vi "Read XNET.vi"(8 "error in":errorcluster, 11 "PCAN in":refnum<class "PCAN.lvclass">) -> (0 "error out":errorcluster, 3 "PCAN out":refnum<class "PCAN.lvclass">)   [LabVIEW 2024, in "PCAN.lvclass"]
uses:
  PCAN.lvclass
  D:/git/HAL/HAL/Configurations/CFG Base/CFG Base.lvclass
  Configurations/CFG Base/CFG Base.lvclass/CFG Base.ctl
  PCAN.lvclass/PCAN.ctl
  <vilib>/xnet/xnet.llb/XNET Frame Type CAN.ctl
  <vilib>/xnet/xnet.llb/XNET Convert (Frame CAN to Signal).vi
  Configurations/CFG Base/CFG Base.lvclass
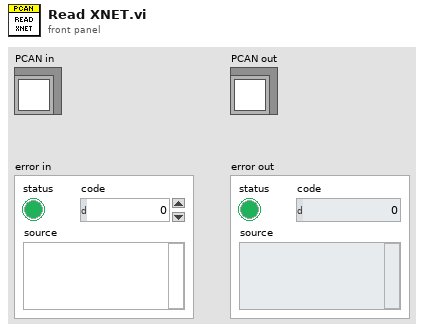
[diagram p1: front panel]
types:
  T1 = typedef "TPCANHandle.ctl" = enum16{"PCAN_NONEBUS  0x000", "PCAN_ISABUS1  0x21", "PCAN_ISABUS2  0x22", "PCAN_ISABUS3  0x23", "PCAN_ISABUS4  0x24", "PCAN_ISABUS5  0x25", "PCAN_ISABUS6  0x26", "PCAN_ISABUS7  0x27", "PCAN_ISABUS8  0x28", "PCAN_DNGBUS1  0x31", "PCAN_PCIBUS1  0x41", "PCAN_PCIBUS1  0x42", "PCAN_PCIBUS1  0x43", "PCAN_PCIBUS1  0x44", "PCAN_PCIBUS1  0x45", "PCAN_PCIBUS1  0x46", "PCAN_PCIBUS1  0x47", "PCAN_PCIBUS1  0x48", "PCAN_PCIBUS1  0x409", "PCAN_PCIBUS1  0x40A", "PCAN_PCIBUS1  0x40B", "PCAN_PCIBUS1  0x40C", "PCAN_PCIBUS1  0x40D", "PCAN_PCIBUS1  0x40E", "PCAN_PCIBUS1  0x40F", "PCAN_PCIBUS1  0x410", "PCAN_USBBUS1  0x51", "PCAN_USBBUS2  0x52", "PCAN_USBBUS3  0x53", "PCAN_USBBUS4  0x54", "PCAN_USBBUS5  0x55", "PCAN_USBBUS6  0x56", "PCAN_USBBUS7  0x57", "PCAN_USBBUS8  0x58", "PCAN_USBBUS9  0x509", "PCAN_USBBUS10  0x50A", "PCAN_USBBUS11  0x50B", "PCAN_USBBUS12  0x50C", "PCAN_USBBUS13  0x50D", "PCAN_USBBUS14  0x50E", "PCAN_USBBUS15  0x50F", "PCAN_USBBUS16  0x510", "PCAN_PCCBUS1  0x61", "PCAN_PCCBUS2  0x62", "PCAN_LANBUS1  0x801", "PCAN_LANBUS2  0x802", "PCAN_LANBUS3  0x803", "PCAN_LANBUS4  0x804", "PCAN_LANBUS5  0x805", "PCAN_LANBUS6  0x806", "PCAN_LANBUS7  0x807", "PCAN_LANBUS8  0x808", "PCAN_LANBUS9  0x809", "PCAN_LANBUS10  0x80A", "PCAN_LANBUS11  0x80B", "PCAN_LANBUS12  0x80C", "PCAN_LANBUS13  0x80D", "PCAN_LANBUS14  0x80E", "PCAN_LANBUS15  0x80F", "PCAN_LANBUS16  0x810"}
  T2 = typedef "TPCANTimestamp.ctl" = cluster{"millis overflow":u16, "millis ":u32, "micros":u16}
  T3 = typedef "CAN MSG Cluster.ctl" = cluster{"ID":u32, "MSG type":u8, "DLC":u8, "DATA":u8[]}
  T4 = typedef "XNET Frame Type CAN.ctl" = u8
  T5 = cluster{"timestamp":timestamp, "payload":u8[], "identifier":u32, "type":T4, "extended?":bool, "echo?":bool}
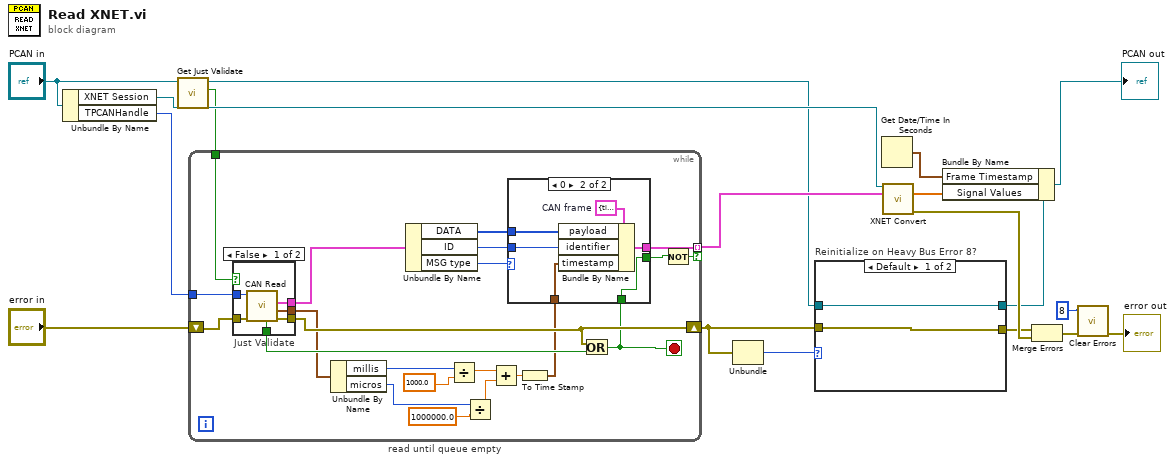
[diagram p0: block diagram]
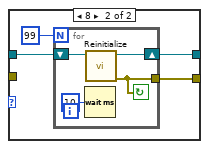
[diagram p2: hidden frame]
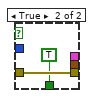
[diagram p3: hidden frame]
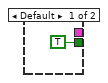
[diagram p4: hidden frame]
diagram:
  n1 = Unbundle By Name("PCAN in") -> ("XNET Session"=w16:refnum<k21>, "TPCANHandle"=w15:T1)
  n2 = call "Get Just Validate.vi"("CFG Base in"="PCAN in") -> ("Just Validate"=w2:bool, "CFG Base out"=w3:refnum<class "PCAN.lvclass">)  [unwired: 9 in]
  n3 = while "read until queue empty" {
    tunnel: w15 -> [w40]
    shift-right: [w37] -> w13
    shift-left: "error in" -> [w39]
    tunnel: [w23] -> w17 mode=indexing if=w36
    tunnel: w2 -> [w19]
    stop <- w20 stop-if-true
    n4 = case "Just Validate" shown="False" w19 {
      tunnel: w40 -> [w46 _]
      tunnel: w39 -> [w45 w48]
      tunnel: [w44 TRUE ("rcv queue empty")] -> w38
      tunnel: [w43 w48] -> w37
      tunnel: [w42 _] -> w35
      tunnel: [w41 _] -> w32
      frame False {
        n5 = call <instrlib>:"CAN Read.vi"("error in (no error)"=w45, "TPCANHandle"=w46) -> ("error out"=w43:errorcluster, "TPCANTimestamp out"=w41:T2, "CAN_Message out"=w42:T3, "rcv queue empty"=w44:bool)  [unwired: 5 in, 1 out]
      }
      frame True {
      }
    }
    n6 = Unbundle By Name(w32) -> ("millis"=w31:u32, "micros"=w29:u16)
    n7 = Unbundle By Name(w35) -> ("DATA"=w34:u8[], "ID"=w33:u32, "MSG type"=w22:u8)
    n8 = Divide(x=w31, y=1000.0) -> (x/y=w25:dbl)
    n9 = Divide(x=w29, y=1000000.0) -> (x/y=w26:dbl)
    n10 = Add(x=w25, y=w26) -> (x+y=w27:dbl)
    n11 = To Time Stamp(1:w27) -> (0:w24:timestamp)
    n12 = Or(x=w37, y=w38) -> (x .or. y?=w20:bool)
    n13 = case shown="0" w22 {
      tunnel: w34 -> [_ w54]
      tunnel: w33 -> [_ w53]
      tunnel: w24 -> [_ w52]
      tunnel: [_ w51] -> w23
      tunnel: [TRUE w50] -> w21
      tunnel: w20 -> [_ w50]
      frame Default {
      }
      frame 0 {
        w55 = T5 {"timestamp"=timestamp(0 s since 1904-01-01), "payload"=[], "identifier"=0, "type"=0, "extended?"=FALSE, "echo?"=FALSE}  # CAN frame
        n14 = Bundle By Name(cluster=w55, "payload"=w54, "identifier"=w53, "timestamp"=w52) -> (w51:T5)
      }
    }
    n15 = Not(x=w21) -> (.not. x?=w36:bool)
  }
  n16 = Unbundle(w13) -> ("code"=w14:i32)  [unwired: 2 out]
  n17 = case "Reinitialize on Heavy Bus Error 8?" shown="Default" w14 {
    tunnel: [w57 w61] -> w11
    tunnel: w13 -> [w57 _]
    tunnel: w3 -> [w56 w60]
    tunnel: [w56 w59] -> w8
    frame Default {
    }
    frame 8 {
      n18 = for {
        N: 99 -> [_]
        tunnel: [w63] -> w61
        shift-right: [w64] -> w59
        shift-left: w60 -> [w65]
        stop <- w63 continue-if-true
        n19 = Wait (ms)(milliseconds to wait=u32 10) -> ()  [unwired: 1 out]
        n20 = call "Reinitialize.vi"("PCAN in"=w65) -> ("error out"=w63:errorcluster, "PCAN out"=w64:refnum<class "PCAN.lvclass">)  [unwired: 9 in]
      }
    }
  }
  n21 = Get Date/Time In Seconds() -> (seconds since 1Jan1904=w1:timestamp)
  n22 = call-poly <vilib>:"XNET Convert.vi"("session in"=w16, "frame data"=w17) -> ("signal data"=w9:dbl[], "error out"=w12:errorcluster)  [unwired: 11 in, 1 out]
  n23 = Bundle By Name(cluster=w8, "Frame Timestamp"=w1, "Signal Values"=w9) -> (→"PCAN out":refnum<class "PCAN.lvclass">)
  n24 = Merge Errors(w11, w12) -> (w10:errorcluster)
  n25 = call <vilib>:"Clear Errors.vi"("error in (no error)"=w10, "specific error code to clear (0: all)"=8) -> ("error out"=→"error out":errorcluster)  [unwired: 4 in, 1 out]
